vi "2D Animation.vi"(0 "Goal":cluster{"x":dbl, "y":dbl}={"x"=nan, "y"=nan}, 1 "2D Pic reference":refnum<vi>, 2 "initialize":bool, 5 "Translation":cluster{"x":dbl, "y":dbl, "z":dbl}, 7 "Rotation":dbl=1.54, 11 "Zoom Factor":sgl(slide)=1.0 scale=0.5..2.0, 12 "cartesian axis attributes":T2={"x minimum"=-10.0, "x maximum"=10.0, "x log?"=FALSE, "x precision"=1, "x format"=enum."Decimal", "y minimum"=-10.0, "y maximum"=10.0, "y log?"=FALSE, "y precision"=1, "y format"=enum."Decimal"}) -> (4 "Map Floor":picture)   [LabVIEW 2017]
uses:
  <vilib>/Utility/miscctls.llb/LVBoundsTypeDef.ctl
  <vilib>/picture/cartesn2.llb/XY Plot Type.ctl
  <vilib>/ptbypt/NI_PtbyPt.lvlib
  <vilib>/picture/picture.llb/imagedata.ctl
panel:
  in  "cartesian axis attributes 2":T1={"x minimum"=-10.0, "x maximum"=10.0, "y minimum"=-10.0, "y maximum"=10.0}
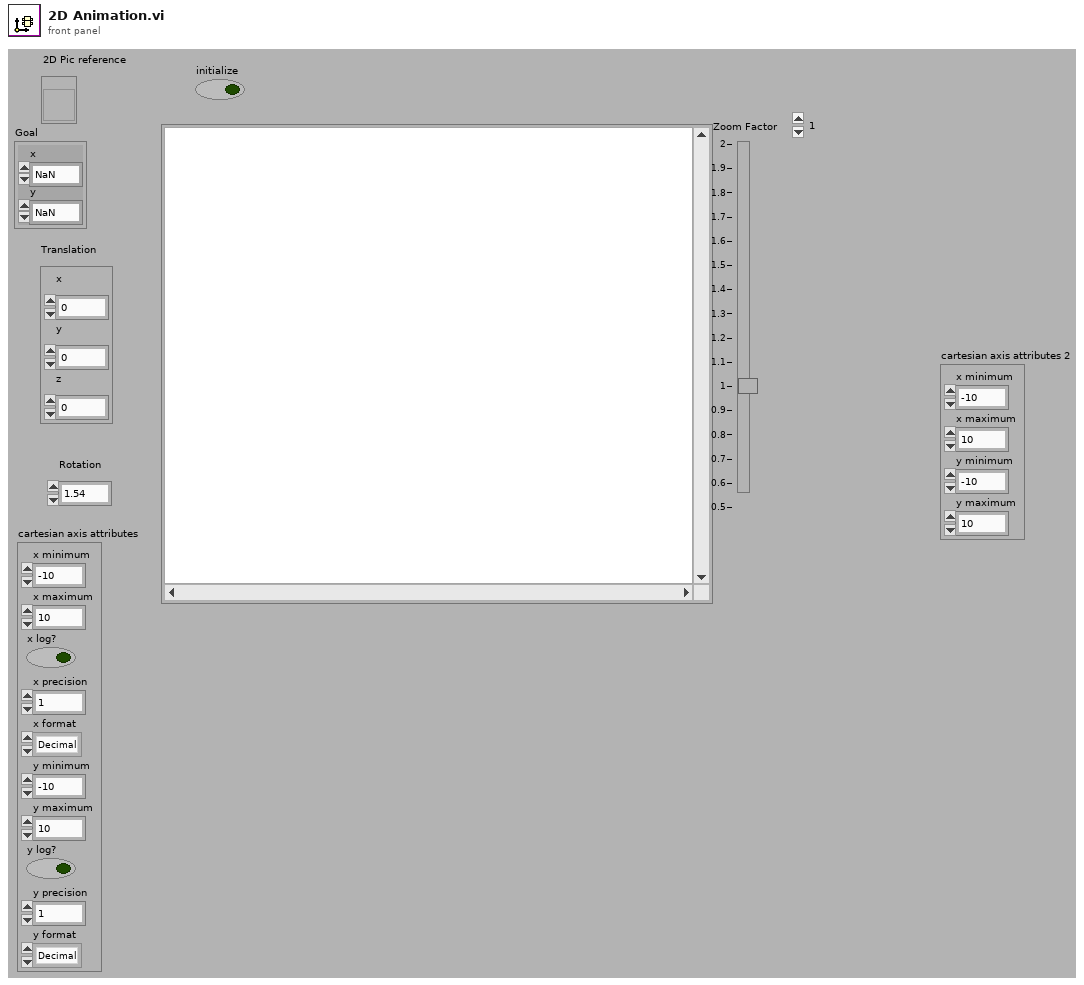
[diagram p1: front panel]
types:
  T1 = cluster{"x minimum":dbl, "x maximum":dbl, "y minimum":dbl, "y maximum":dbl}
  T2 = cluster{"x minimum":dbl, "x maximum":dbl, "x log?":bool, "x precision":u8, "x format":enum8{"Decimal", "Scientific", "Engineering", "Binary", "Octal", "Hex"}, "y minimum":dbl, "y maximum":dbl, "y log?":bool, "y precision":u8, "y format":enum8{"Decimal", "Scientific", "Engineering", "Binary", "Octal", "Hex"}}
  T3 = cluster{"Width":u16, "Style":enum32{"Solid", "Dash", "Dot", "DashDot", "DashDotDot"}}
  T4 = typedef "LVBoundsTypeDef.ctl" = cluster{"Width":u32, "Height":u32}
  T5 = typedef "imagedata.ctl" = cluster{"image type":i32, "image depth":i32, "image":u8[], "mask":u8[], "colors":u32[], "Rectangle":cluster{"left":i16, "top":i16, "right":i16, "bottom":i16}}
  T6 = typedef "XY Plot Type.ctl" = enum16{"points", "squares", "circles", "connected points", "connected squares", "connected circles", "comb plot", "sized scatter plot", "sized-colored scatter plot", "min-max lines"}
  T7 = cluster{"plot color":u32, "XY plot type":T6, "baseline":dbl}
  T8 = cluster{"min size":i16, "max size":i16, "maps to max size":i16, "color array":u32[]}
  T9 = cluster{"line color":u32, "text color":u32, "tick length(3)":i16, "crossing axes":bool, "visible grid?":bool}
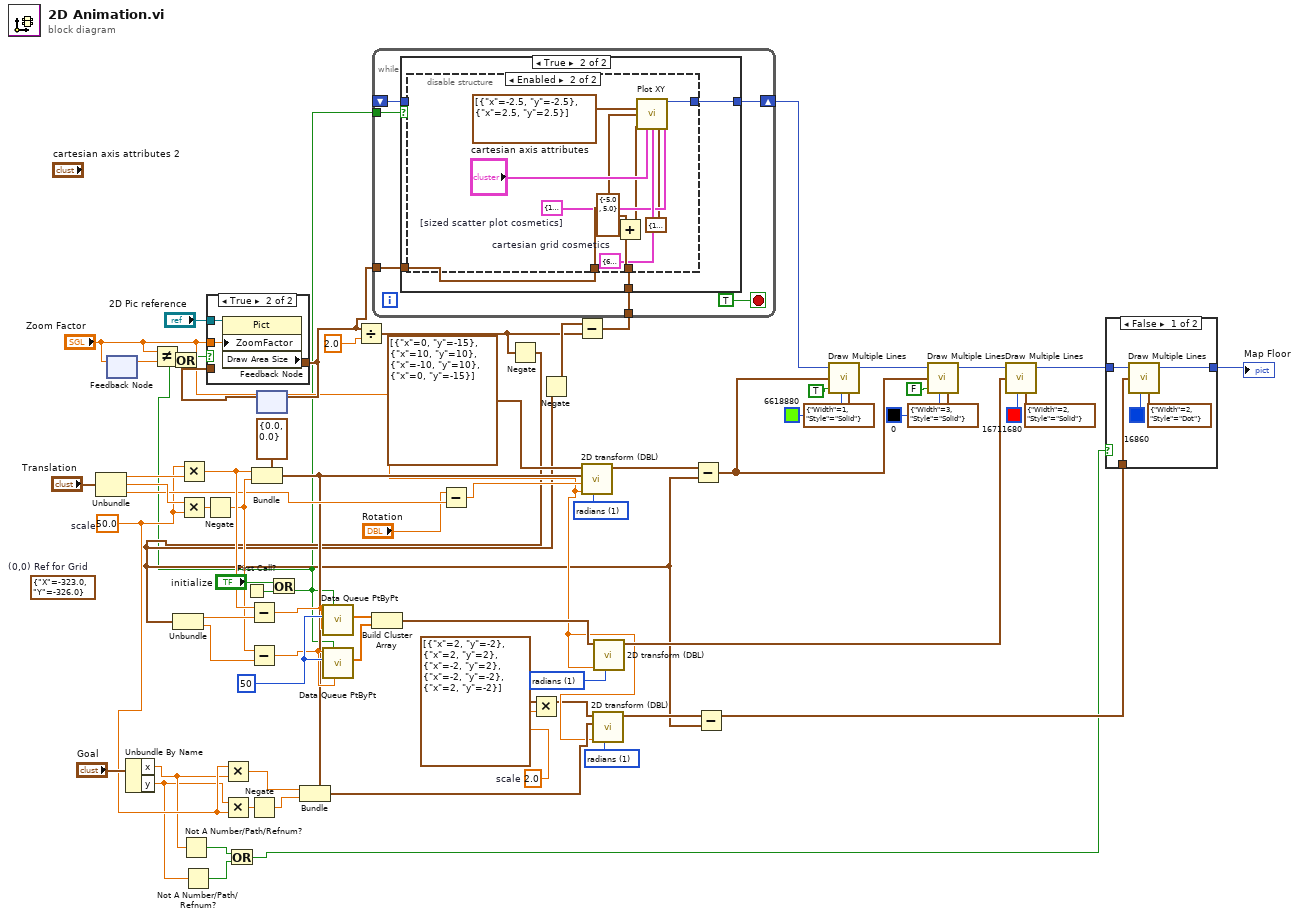
[diagram p0: block diagram]
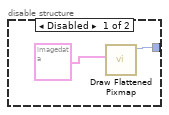
[diagram p4: hidden frame]
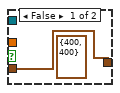
[diagram p5: hidden frame]
diagram:
  w8 = 2.0  # scale
  w24 = u16 1 items=["degree", "radians"] ("angle unit")
  w28 = u16 1 items=["degree", "radians"] ("angle unit")
  w47 = u16 1 items=["degree", "radians"] ("angle unit")
  (unwired) cluster{"X":dbl, "Y":dbl} {"X"=-323.0, "Y"=-326.0}  # (0,0) Ref for Grid
  w17 = 50.0  # scale
  w57 = 50 ("sample length")
  n1 = Unbundle("Translation") -> ("x"=w61:dbl, "y"=w62:dbl, "z"=w37:dbl)
  n2 = feedback #1() -> (w55:sgl)  [unwired: 1 in]
  n3 = feedback-in #1("Zoom Factor") -> ()
  n4 = Unbundle By Name("Goal") -> ("x"=w7:dbl, "y"=w6:dbl)
  n5 = Not Equal?(x="Zoom Factor", y=w55) -> (x != y?=w56:bool)
  n6 = Multiply(x=w17, y=w61) -> (x*y=w52:dbl)
  n7 = Multiply(x=w62, y=w17) -> (x*y=w66:dbl)
  n8 = Not A Number/Path/Refnum?(number/path/refnum=w7) -> (NaN/Path/Refnum?=w4:bool)
  n9 = Not A Number/Path/Refnum?(number/path/refnum=w6) -> (NaN/Path/Refnum?=w5:bool)
  n10 = Negate(x=w66) -> (-x=w46:dbl)
  n11 = Multiply(x=w17, y=w7) -> (x*y=w15:dbl)
  n12 = Multiply(x=w6, y=w17) -> (x*y=w19:dbl)
  n13 = Or(x=w4, y=w5) -> (x .or. y?=w3:bool)
  n14 = First Call?() -> (First Call?: T/F=w45:bool)
  n15 = Negate(x=w19) -> (-x=w16:dbl)
  n16 = Bundle(cluster=cluster{"x":dbl, "y":dbl} {"x"=0.0, "y"=0.0}, "x"=w52, "y"=w46) -> (w14:cluster{"x":dbl, "y":dbl})
  n17 = feedback #2() -> (w26:T4)  [unwired: 1 in]
  n18 = Or(x="initialize", y=w45) -> (x .or. y?=w1:bool)
  n19 = Or(x=w56, y=w1) -> (x .or. y?=w2:bool)
  n20 = case shown="True" w2 {
    tunnel: "Zoom Factor" -> [_ w74]
    tunnel: "2D Pic reference" -> [_ w73]
    tunnel: [w71 w72] -> w27
    tunnel: w26 -> [w71 _]
    frame False {
      (unwired) T4 {"Width"=400, "Height"=400} ("Draw Area Size")
    }
    frame True {
      n21 = property on="Property Node" class="Pict"(reference=w73, "ZoomFactor"=w74) -> ("Draw Area Size"=w72:T4)  [unwired: 1 in, 2 out]
    }
  }
  n22 = feedback-in #2(w27) -> ()
  n23 = Bundle(cluster=w14, "x"=w15, "y"=w16) -> (w13:cluster{"x":dbl, "y":dbl})
  n24 = Divide(x=w27, y=2.0 ("x")) -> (x/y=w25:cluster{"Width":dbl, "Height":dbl})
  n25 = Subtract(x="Rotation", y=w37) -> (x-y=w36:dbl)
  n26 = Negate(x=w25) -> (-x=w10:cluster{"Width":dbl, "Height":dbl})
  n27 = Unbundle(w10) -> ("Width"=w59:dbl, "Height"=w60:dbl)
  n28 = Subtract(x=w52, y=w59) -> (x-y=w38:dbl)
  n29 = Subtract(x=w46, y=w60) -> (x-y=w39:dbl)
  n30 = call <vilib>:"Data Queue PtByPt.vi"("initial queue element"=w38, "initialize"=w1, "sample length"=w57, "input data point"=w38) -> ("Current Queue"=w51:dbl[])  [unwired: 3 in, 4 out]
  n31 = call <vilib>:"Data Queue PtByPt.vi"("initial queue element"=w39, "initialize"=w1, "sample length"=w57, "input data point"=w39) -> ("Current Queue"=w58:dbl[])  [unwired: 3 in, 4 out]
  n32 = Build Cluster Array(w51, w58) -> (w30:cluster{dbl, dbl}[])
  n33 = Multiply(x=cluster{"x":i16, "y":i16}[] [{"x"=2, "y"=-2}, {"x"=2, "y"=2}, {"x"=-2, "y"=2}, {"x"=-2, "y"=-2}, {"x"=2, "y"=-2}] ("line endpoints"), y=w8) -> (x*y=w9:cluster{"x":dbl, "y":dbl}[])
  n34 = Negate(x=w10) -> (-x=w32:cluster{"Width":dbl, "Height":dbl})
  n35 = Subtract(x=w32, y=w25) -> (x-y=w31:cluster{"Width":dbl, "Height":dbl})
  n36 = while {
    shift-right: [w80] -> w44
    shift-left: _ -> [w78]
    tunnel: w1 -> [w79]
    tunnel: w31 -> [w76]
    tunnel: w27 -> [w75]
    stop <- TRUE stop-if-true
    n37 = case shown="True" w79 {
      tunnel: [w81 w84] -> w80
      tunnel: w78 -> [w81 _]
      tunnel: w76 -> [_ w83]
      tunnel: w75 -> [_ w82]
      frame False {
      }
      frame True {
        n38 = disable-structure shown="Enabled" {
          disable-tunnel: [w86 w96] -> w84
          disable-tunnel: w83 -> [_ w94]
          disable-tunnel: w82 -> [_ w91]
          frame Disabled {
            n39 = call <vilib>:"Draw Flattened Pixmap.vi"("image data"=T5 {"image type"=0, "image depth"=24, "image"=array[1269282 elements], "mask"=[], "colors"=[], "Rectangle"={"left"=0, "top"=0, "right"=658, "bottom"=643}}) -> ("new picture"=w86:picture)  [unwired: 8 in]
          }
          frame Enabled {
            w90 = T8 {"min size"=1, "max size"=5, "maps to max size"=5, "color array"=[16777216, 65280, 16711680, 255]}  # [sized scatter plot cosmetics]
            w92 = T9 {"line color"=6710886, "text color"=13421772, "tick length(3)"=3, "crossing axes"=FALSE, "visible grid?"=TRUE}  # cartesian grid cosmetics
            n40 = Add(x=w94, y=cluster{"Width":dbl, "Height":dbl} {"Width"=-5.0, "Height"=5.0} ("x")) -> (x+y=w88:cluster{"Width":dbl, "Height":dbl})
            n41 = call <vilib>:"Plot XY.vi"("data"=cluster{"x":dbl, "y":dbl}[] [{"x"=-2.5, "y"=-2.5}, {"x"=2.5, "y"=2.5}], "dimensions (w,h)"=w91, "top left point(0, 0)"=w88, "cartesian axis attributes"="cartesian axis attributes", "cartesian grid cosmetics"=w92, "XY plot cosmetics"=T7 {"plot color"=16777216, "XY plot type"=enum."connected points", "baseline"=0.0}, "[sized scatter plot cosmetics]"=w90) -> ("new picture"=w96:picture)  [unwired: 8 in]
          }
        }
      }
    }
  }
  n42 = call "2D transform (DBL).vi"("angle unit"=w47, "Scale"="Zoom Factor", "Rotation Angle"=w36, "Translation"=w14, "line endpoints"=cluster{"x":i16, "y":i16}[] [{"x"=0, "y"=-15}, {"x"=10, "y"=10}, {"x"=-10, "y"=10}, {"x"=0, "y"=-15}]) -> ("tranformed line endpoint"=w48:cluster{"x":dbl, "y":dbl}[])  [unwired: 6 in]
  n43 = call "2D transform (DBL).vi"("angle unit"=w24, "Scale"="Zoom Factor", "Translation"=w13, "line endpoints"=w9) -> ("tranformed line endpoint"=w21:cluster{"x":dbl, "y":dbl}[])  [unwired: 7 in]
  n44 = call "2D transform (DBL).vi"("angle unit"=w28, "Scale"="Zoom Factor", "line endpoints"=w30) -> ("tranformed line endpoint"=w29:cluster{"x":dbl, "y":dbl}[])  [unwired: 8 in]
  n45 = Subtract(x=w48, y=w10) -> (x-y=w40:cluster{dbl, dbl}[])
  n46 = Subtract(x=w21, y=w10) -> (x-y=w11:cluster{dbl, dbl}[])
  n47 = call <vilib>:"Draw Multiple Lines.vi"("picture"=w44, "line endpoints"=w40, "fill?(F)"=TRUE, "color(black)"=u32 6618880, "pen"=T3 {"Width"=1, "Style"=enum."Solid"}) -> ("new picture"=w68:picture)  [unwired: 4 in]
  n48 = call <vilib>:"Draw Multiple Lines.vi"("picture"=w68, "line endpoints"=w40, "fill?(F)"=FALSE, "color(black)"=u32 0, "pen"=T3 {"Width"=3, "Style"=enum."Solid"}) -> ("new picture"=w50:picture)  [unwired: 4 in]
  n49 = call <vilib>:"Draw Multiple Lines.vi"("picture"=w50, "line endpoints"=w29, "color(black)"=u32 16711680, "pen"=T3 {"Width"=2, "Style"=enum."Solid"}) -> ("new picture"=w23:picture)  [unwired: 5 in]
  n50 = case shown="False" w3 {
    tunnel: w23 -> [w99 w102]
    tunnel: [w98 w102] -> w22
    tunnel: w11 -> [w97 _]
    frame False {
      n51 = call <vilib>:"Draw Multiple Lines.vi"("picture"=w99, "line endpoints"=w97, "color(black)"=u32 16860, "pen"=T3 {"Width"=2, "Style"=enum."Dot"}) -> ("new picture"=w98:picture)  [unwired: 5 in]
    }
    frame True {
    }
  }
  "Map Floor" <- w22
